vi "方框循环2.vi"() -> ()   [LabVIEW 2018]
panel:
  in  "y运动速度（步数/s":i32=200
  in  "y运动加速度":i32=200
  in  "停止循环":bool
  in  "循环次数":i32=20
  in  "x运动加速度":i32=200
  out "error out":errorcluster
  in  "停止程序":bool
  in  "y距离/um":dbl=2.0
  in  "y比例(um/步)":dbl=0.14
  in  "x距离/um":dbl=2.0
  in  "x比例(um/步)":dbl=0.048
  in  "开始移动":bool
  in  "x运动速度（步数/s）":i32=200
  out "DeviceKey Out":string
  out "Identification":string
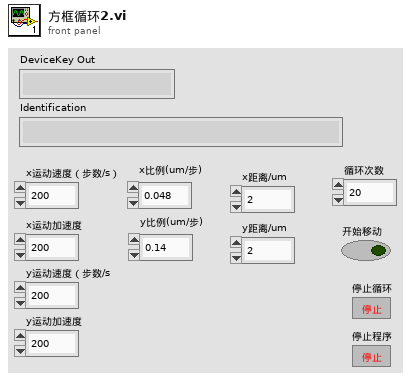
[diagram p1: front panel]
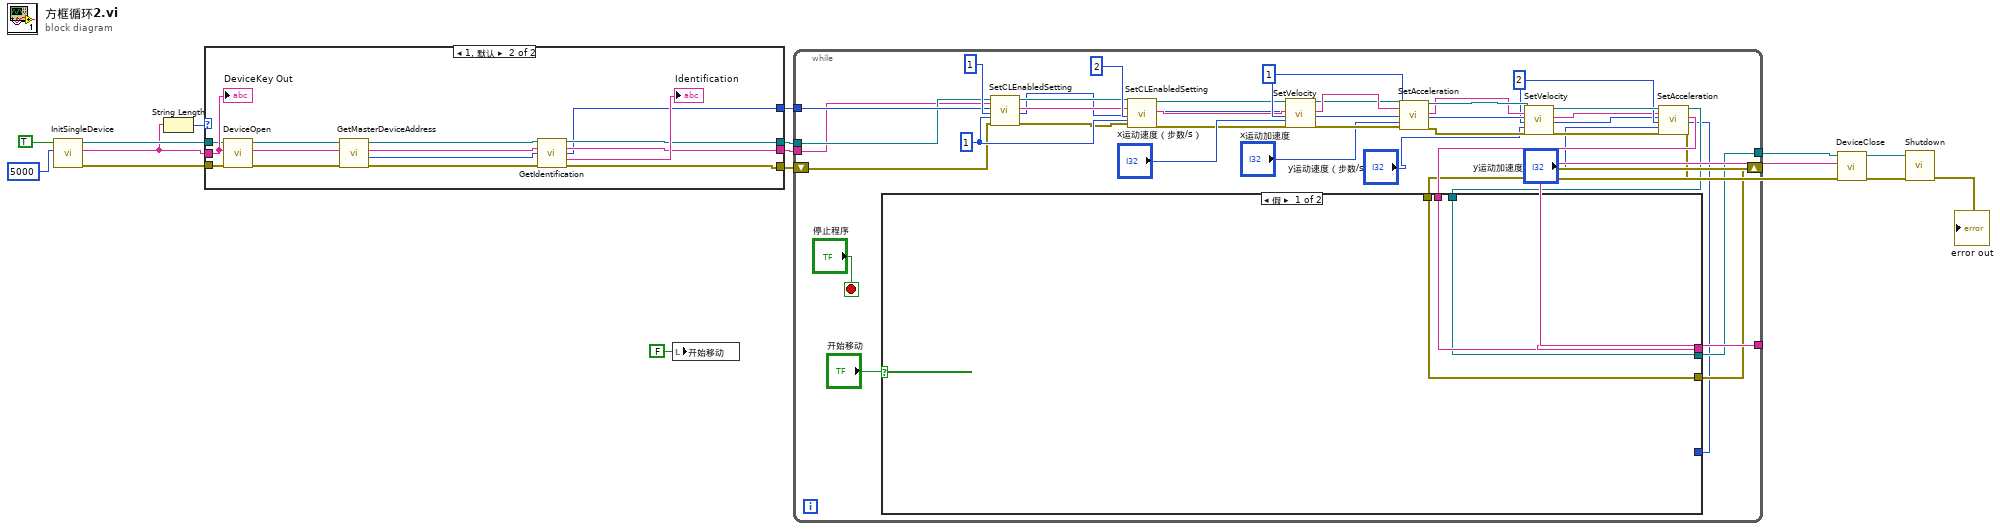
[diagram p0: block diagram]
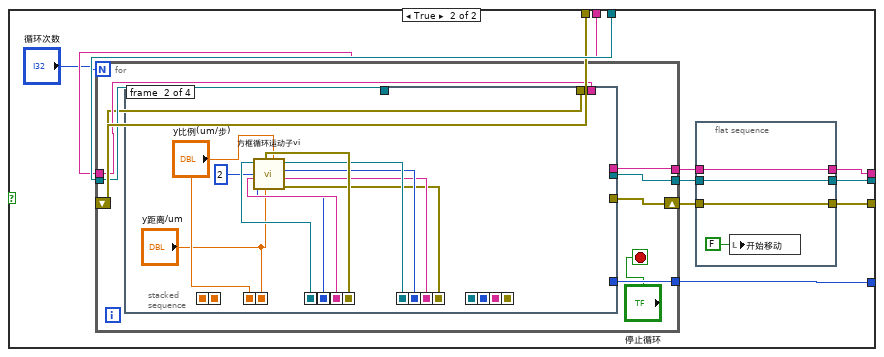
[diagram p2: hidden frame]
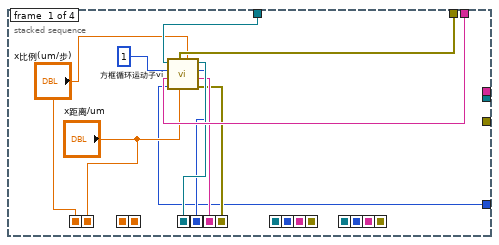
[diagram p3: hidden frame]
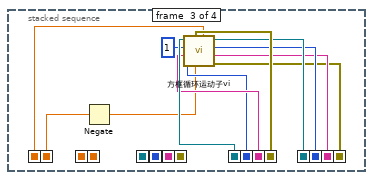
[diagram p4: hidden frame]
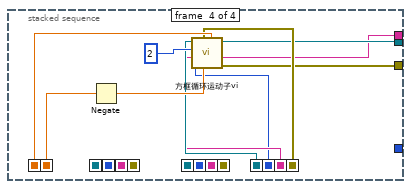
[diagram p5: hidden frame]
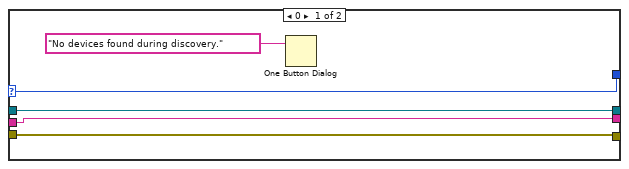
[diagram p6: hidden frame]
diagram:
  n1 = call "InitSingleDevice.vi"("msecDelayForDiscovery"=5000, "logging"=TRUE) -> ("error out"=w13:errorcluster, "DeviceKey Out"=w12:string, "CmdLib Out"=w14:refnum<k24>)  [unwired: 3 in]
  n2 = String Length(string=w12) -> (length=w15:i32)
  n3 = case shown="1, 默认" w15 {
    selector: w15 -> [w18 _]
    tunnel: w14 -> [w21 w28]
    tunnel: w13 -> [w20 w32]
    tunnel: w12 -> [w19 w30]
    tunnel: [w21 w26] -> w10
    tunnel: [w20 w25] -> w8
    tunnel: [w19 w24] -> w9
    tunnel: [w18 w23] -> w11
    frame 0 {
      n4 = One Button Dialog(message="No devices found during discovery.") -> ()  [unwired: 1 in, 1 out]
    }
    frame 1, Default {
      n5 = call "DeviceOpen.vi"("error in (no error)"=w32, "DeviceKey In"=w30, "CmdLib In"=w28) -> ("error out"=w31:errorcluster, "DeviceKey Out"=w29:string, "CmdLib Out"=w27:refnum<k24>)  [unwired: 2 in]
      n6 = call "GetMasterDeviceAddress.vi"("error in (no error)"=w31, "DeviceKey In"=w29, "CmdLib In"=w27) -> ("error out"=w35:errorcluster, "Device Address"=w36:i32, "DeviceKey Out"=w33:string, "CmdLib Out"=w34:refnum<k24>)  [unwired: 1 in]
      n7 = call "GetIdentification.vi"("CmdLib In"=w34, "DeviceKey In"=w33, "Device Address In"=w36, "error in (no error)"=w35) -> ("CmdLib Out"=w26:refnum<k24>, "DeviceKey Out"=w24:string, "Device Address Out"=w23:i32, "Identification"=→"Identification":string, "error out"=w25:errorcluster)  [unwired: 7 in]
      "DeviceKey Out" <- w30
    }
  }
  n8 = local write "开始移动"(FALSE ("开始移动")) -> ()
  n9 = while {
    tunnel: w11 -> [w76]
    tunnel: w10 -> [w75]
    tunnel: w9 -> [w74]
    shift-right: [w66] -> w4
    shift-left: w8 -> [w73]
    tunnel: [w65] -> w3
    tunnel: [w64] -> w2
    stop <- "停止程序" stop-if-true
    w52 = 2
    w62 = 1
    w78 = 1 ("Setting")
    n10 = call "SetCLEnabledSetting.vi"("CmdLib In"=w75, "DeviceKey In"=w74, "Device Address In"=w76, "Motor"=1, "Setting"=w78, "error in (no error)"=w73) -> ("CmdLib Out"=w72:refnum<k24>, "DeviceKey Out"=w71:string, "Device Address Out"=w70:i32, "error out"=w69:errorcluster)  [unwired: 10 in]
    n11 = call "SetCLEnabledSetting.vi"("CmdLib In"=w72, "DeviceKey In"=w71, "Device Address In"=w70, "Motor"=2, "Setting"=w78, "error in (no error)"=w69) -> ("CmdLib Out"=w49:refnum<k24>, "DeviceKey Out"=w46:string, "Device Address Out"=w45:i32, "error out"=w44:errorcluster)  [unwired: 10 in]
    n12 = call "SetVelocity.vi"("CmdLib In"=w49, "DeviceKey In"=w46, "Device Address In"=w45, "Motor"=w62, "Steps Per Sec"="x运动速度（步数/s）", "error in (no error)"=w44) -> ("CmdLib Out"=w59:refnum<k24>, "DeviceKey Out"=w60:string, "Device Address Out"=w63:i32, "error out"=w61:errorcluster)  [unwired: 10 in]
    n13 = call "SetAcceleration.vi"("CmdLib In"=w59, "DeviceKey In"=w60, "Device Address In"=w63, "Motor"=w62, "Steps Per Sec 2"="x运动加速度", "error in (no error)"=w61) -> ("CmdLib Out"=w58:refnum<k24>, "DeviceKey Out"=w57:string, "Device Address Out"=w56:i32, "error out"=w55:errorcluster)  [unwired: 10 in]
    n14 = call "SetVelocity.vi"("CmdLib In"=w58, "DeviceKey In"=w57, "Device Address In"=w56, "Motor"=w52, "Steps Per Sec"="y运动速度（步数/s", "error in (no error)"=w55) -> ("CmdLib Out"=w53:refnum<k24>, "DeviceKey Out"=w50:string, "Device Address Out"=w51:i32, "error out"=w54:errorcluster)  [unwired: 10 in]
    n15 = call "SetAcceleration.vi"("CmdLib In"=w53, "DeviceKey In"=w50, "Device Address In"=w51, "Motor"=w52, "Steps Per Sec 2"="y运动加速度", "error in (no error)"=w54) -> ("CmdLib Out"=w43:refnum<k24>, "DeviceKey Out"=w42:string, "Device Address Out"=w40:i32, "error out"=w41:errorcluster)  [unwired: 10 in]
    n16 = case shown="假" "开始移动" {
      tunnel: w43 -> [w80 w93]
      tunnel: w42 -> [w81 w92]
      tunnel: w40 -> [_ w91]
      tunnel: w41 -> [w82 w90]
      tunnel: [w80 w84] -> w64
      tunnel: [w81 w83] -> w65
      tunnel: [w82 w85] -> w66
      frame False {
      }
      frame True {
        n17 = for {
          N: "循环次数" -> [_]
          tunnel: w91 -> [w102]
          shift-right: [w99] -> w86
          shift-left: w90 -> [w103]
          tunnel: w93 -> [w105]
          tunnel: w92 -> [w104]
          tunnel: [w101] -> w88
          tunnel: [w100] -> w87
          stop <- "停止循环" stop-if-true
          n18 = stacked-sequence {
            seq-local: [w112 _ _ _] -> [_ w127 _ _]
            seq-local: [w111 _ _ _] -> [_ w125 _ _]
            seq-local: [w110 _ _ _] -> [_ w126 _ _]
            seq-local: [w109 _ _ _] -> [_ w124 _ _]
            seq-local: [_ w122 _ _] -> [_ _ w139 _]
            seq-local: [_ w121 _ _] -> [_ _ w136 _]
            seq-local: [_ w120 _ _] -> [_ _ w137 _]
            seq-local: [_ w119 _ _] -> [_ _ w135 _]
            seq-local: ["x比例(um/步)" _ _ _] -> [_ _ w134 _]
            seq-local: ["x距离/um" _ _ _] -> [_ _ w133 _]
            seq-local: [_ "y比例(um/步)" _ _] -> [_ _ _ w150]
            seq-local: [_ "y距离/um" _ _] -> [_ _ _ w149]
            seq-local: [_ _ w131 _] -> [_ _ _ w146]
            seq-local: [_ _ w130 _] -> [_ _ _ w144]
            seq-local: [_ _ w129 _] -> [_ _ _ w145]
            seq-local: [_ _ w128 _] -> [_ _ _ w143]
            tunnel: w105 -> [w116 _ _ _]
            tunnel: w104 -> [w115 _ _ _]
            tunnel: w103 -> [w114 _ _ _]
            tunnel: [_ _ _ w142] -> w100
            tunnel: [_ _ _ w141] -> w101
            tunnel: [_ _ _ w140] -> w99
            tunnel: w102 -> [w106 _ _ _]
            frame #0 {
              n19 = call "方框循环运动子vi.vi"("比例(um/步)"="x比例(um/步)", "运行步数/um"="x距离/um", "error in (no error)"=w114, "Device Address In"=w106, "DeviceKey In"=w115, "Motor"=1, "CmdLib In"=w116) -> ("error out"=w109:errorcluster, "DeviceKey Out"=w110:string, "Device Address Out"=w111:i32, "CmdLib Out"=w112:refnum<k24>)  [unwired: 1 in]
            }
            frame #1 {
              n20 = call "方框循环运动子vi.vi"("比例(um/步)"="y比例(um/步)", "运行步数/um"="y距离/um", "error in (no error)"=w124, "Device Address In"=w125, "DeviceKey In"=w126, "Motor"=2, "CmdLib In"=w127) -> ("error out"=w119:errorcluster, "DeviceKey Out"=w120:string, "Device Address Out"=w121:i32, "CmdLib Out"=w122:refnum<k24>)  [unwired: 1 in]
            }
            frame #2 {
              n21 = Negate(x=w133) -> (-x=w132:dbl)
              n22 = call "方框循环运动子vi.vi"("比例(um/步)"=w134, "运行步数/um"=w132, "error in (no error)"=w135, "Device Address In"=w136, "DeviceKey In"=w137, "Motor"=1, "CmdLib In"=w139) -> ("error out"=w128:errorcluster, "DeviceKey Out"=w129:string, "Device Address Out"=w130:i32, "CmdLib Out"=w131:refnum<k24>)  [unwired: 1 in]
            }
            frame #3 {
              n23 = Negate(x=w149) -> (-x=w148:dbl)
              n24 = call "方框循环运动子vi.vi"("比例(um/步)"=w150, "运行步数/um"=w148, "error in (no error)"=w143, "Device Address In"=w144, "DeviceKey In"=w145, "Motor"=2, "CmdLib In"=w146) -> ("error out"=w140:errorcluster, "DeviceKey Out"=w141:string, "CmdLib Out"=w142:refnum<k24>)  [unwired: 1 in, 1 out]
            }
          }
        }
        n25 = flat-sequence {
          tunnel: w88 -> [w94]
          tunnel: w87 -> [w95]
          tunnel: w86 -> [w96]
          tunnel: [w96] -> w85
          tunnel: [w95] -> w84
          tunnel: [w94] -> w83
          frame #0 {
            n26 = local write "开始移动"(FALSE ("开始移动")) -> ()
          }
        }
      }
    }
  }
  n27 = call "DeviceClose.vi"("error in (no error)"=w4, "DeviceKey In"=w3, "CmdLib In"=w2) -> ("error out"=w6:errorcluster, "CmdLib Out"=w7:refnum<k24>)  [unwired: 2 in, 1 out]
  n28 = call "Shutdown.vi"("error in (no error)"=w6, "CmdLib In"=w7) -> ("error out"=→"error out":errorcluster)  [unwired: 4 in, 1 out]
